vi "SubVI_SpeedLimitMsgBW_Auto.vi"(11 "speed":string) -> (3 "limited speed":dbl)   [LabVIEW 2017]
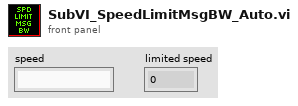
[diagram p1: front panel]
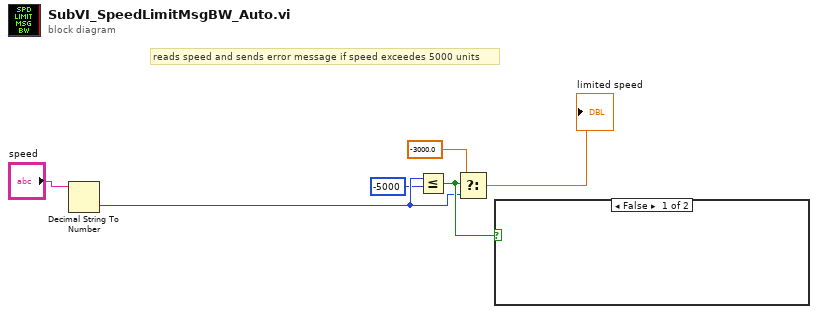
[diagram p0: block diagram]
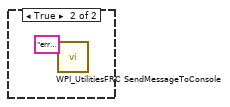
[diagram p2: hidden frame]
diagram:
  # "reads speed and sends error message if speed exceedes 5000 units"
  n1 = Decimal String To Number(string="speed") -> (number=w2:i32)  [unwired: 2 in, 1 out]
  n2 = Less Or Equal?(x=w2, y=-5000) -> (x <= y?=w3:bool)
  n3 = Select(t=-3000.0, s=w3, f=w2) -> (s? t:f=→"limited speed":dbl)
  n4 = case shown="False" w3 {
    frame False {
    }
    frame True {
      n5 = call <vilib>:"WPI_UtilitiesFRC SendMessageToConsole.vi"("Message"="error your speed has exceeded 5000 and is being blocked by autonomous independent VI") -> ()  [unwired: 14 in, 1 out]
    }
  }
